vi "Read Gear Operation.vi"(8 "Command Info":T4) -> (0 "Command Info":T4, 1 "SubSystem Data":T1)   [LabVIEW 2015]
uses:
  <vilib>/Rock Robotics/WPI/Framework/Command Status Info.ctl
  <vilib>/Rock Robotics/WPI/Framework/Completion Status.ctl
  <vilib>/Rock Robotics/WPI/Framework/Completion Notifier.ctl
  Implementation/Gear Setpoints.ctl
  Implementation/Gear Operations.ctl
  Implementation/Gear.ctl
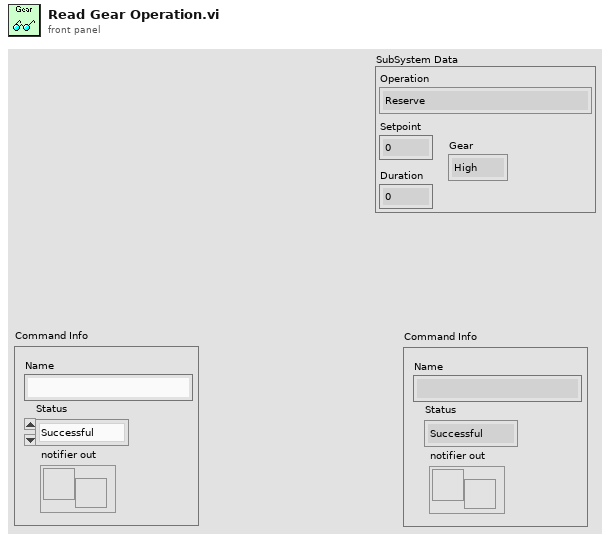
[diagram p1: front panel]
types:
  T1 = typedef "Gear Setpoints.ctl" = cluster{"Operation":T2, "Setpoint":dbl, "Duration":dbl, "Gear":T3}
  T2 = typedef "Gear Operations.ctl" = enum16{"Reserve", "Read Current", "Immediate", "Change Gear"}
  T3 = typedef "Gear.ctl" = enum16{"High", "Low"}
  T4 = typedef "Command Status Info.ctl" = cluster{"Name":string, "Status":T5, "notifier out":T6}
  T5 = typedef "Completion Status.ctl" = enum16{"Successful", "Aborted", "Incomplete"}
  T6 = typedef "Completion Notifier.ctl" = refnum<notifier>
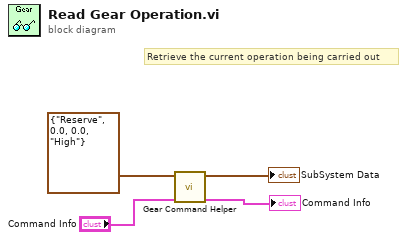
[diagram p0: block diagram]
diagram:
  # "Retrieve the current operation being carried out"
  n1 = call "Gear Command Helper.vi"("Command Info In"="Command Info", "SubSystem Data"=T1 {"Operation"=enum."Reserve", "Setpoint"=0.0, "Duration"=0.0, "Gear"=enum."High"}) -> ("Command Info Out"=→"Command Info":T4, "SubSystem Data"=→"SubSystem Data":T1)  [unwired: 8 in]
